vi "RecursiveLoadInheritance.vi"(7 "TopLevelParentTag":string, 9 "TreeControl":refnum<vi>, 10 "Class":refnum<vi>) -> (2 "ParentName":string)   [LabVIEW 2014, in "ClassInheritanceEditor.lvlib" / "ClassInheritanceEditor.lvclass"]
uses:
  ClassInheritanceEditor.lvclass
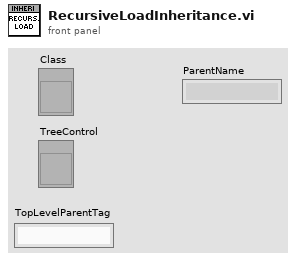
[diagram p1: front panel]
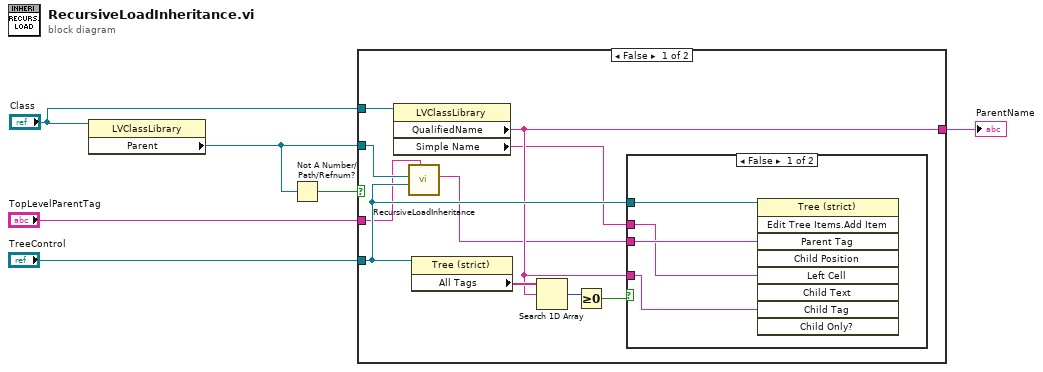
[diagram p0: block diagram]
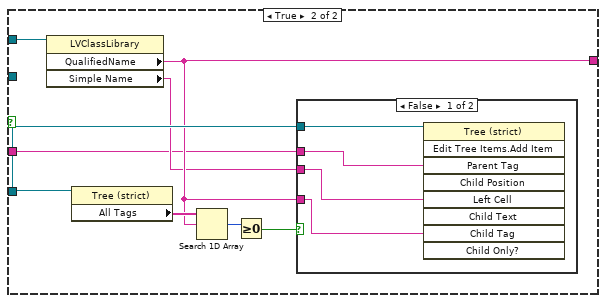
[diagram p3: hidden frame]
diagram:
  n1 = property class="LVClassLibrary"(reference="Class") -> ("Parent"=w5:refnum<vi>)  [unwired: 1 in, 2 out]
  n2 = Not A Number/Path/Refnum?(number/path/refnum=w5) -> (NaN/Path/Refnum?=w6:bool)
  n3 = case shown="False" w6 {
    tunnel: w5 -> [w9 _]
    tunnel: [w12 w24] -> w2
    tunnel: "TreeControl" -> [w13 w27]
    tunnel: "Class" -> [w16 w28]
    tunnel: "TopLevelParentTag" -> [w7 w21]
    frame False {
      n4 = property class="LVClassLibrary"(reference=w16) -> ("QualifiedName"=w12:string, "Simple Name"=w8:string)  [unwired: 1 in, 2 out]
      n5 = call "RecursiveLoadInheritance.vi"("TopLevelParentTag"=w7, "TreeControl"=w13, "Class"=w9) -> ("ParentName"=w10:string)  [unwired: 8 in]
      n6 = property class="Tree (strict)"(reference=w13) -> ("All Tags"=w15:string[])  [unwired: 1 in, 2 out]
      n7 = Search 1D Array(1D array=w15, element=w12) -> (index of element=w14:i32)  [unwired: 1 in]
      n8 = Greater Or Equal To 0?(x=w14) -> (x >= 0?=w11:bool)
      n9 = case shown="False" w11 {
        tunnel: w10 -> [w20 _]
        tunnel: w13 -> [w19 _]
        tunnel: w12 -> [w18 _]
        tunnel: w8 -> [w17 _]
        frame False {
          n10 = invoke on="Invoke Node" class="Tree (strict)" method="Edit Tree Items.Add Item"(reference=w19, "Parent Tag"=w20, "Left Cell"=w17, "Child Tag"=w18) -> ()  [unwired: 5 in, 9 out]
        }
        frame True {
        }
      }
    }
    frame True {
      n11 = property class="LVClassLibrary"(reference=w28) -> ("QualifiedName"=w24:string, "Simple Name"=w22:string)  [unwired: 1 in, 2 out]
      n12 = property class="Tree (strict)"(reference=w27) -> ("All Tags"=w26:string[])  [unwired: 1 in, 2 out]
      n13 = Search 1D Array(1D array=w26, element=w24) -> (index of element=w25:i32)  [unwired: 1 in]
      n14 = Greater Or Equal To 0?(x=w25) -> (x >= 0?=w23:bool)
      n15 = case shown="False" w23 {
        tunnel: w27 -> [w32 _]
        tunnel: w24 -> [w31 _]
        tunnel: w22 -> [w30 _]
        tunnel: w21 -> [w29 _]
        frame False {
          n16 = invoke on="Invoke Node" class="Tree (strict)" method="Edit Tree Items.Add Item"(reference=w32, "Parent Tag"=w29, "Left Cell"=w30, "Child Tag"=w31) -> ()  [unwired: 5 in, 9 out]
        }
        frame True {
        }
      }
    }
  }
  "ParentName" <- w2
